vi "UseArrayOfClusterWithClasses.vi"(9 "Numeric 3":dbl=33.0, 10 "Numeric 2":dbl=22.0, 11 "Numeric":dbl=11.0) -> (3 "output array":T1(array[cluster]))   [LabVIEW 2013]
uses:
  ClassDefinitions/SimpleClassWithProperties/myClass.lvclass
panel:
  in  "array":T1(array[cluster])
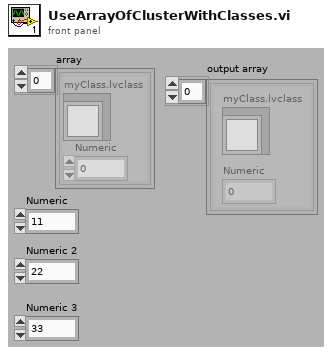
[diagram p1: front panel]
types:
  T1 = cluster{"myClass.lvclass":refnum<class "myClass.lvclass">, "Numeric":dbl}[]
  T2 = cluster{"myClass.lvclass":refnum<class "myClass.lvclass">, "Numeric":dbl}
  T3 = cluster{"myClass.lvclass":refnum<class "myClass.lvclass">, "Numeric 2":dbl}
  T4 = cluster{"myClass.lvclass":refnum<class "myClass.lvclass">, "Numeric 3":dbl}
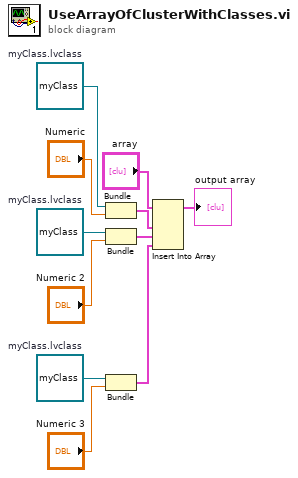
[diagram p0: block diagram]
diagram:
  w1 = refnum<class "myClass.lvclass"> refnum  # myClass.lvclass
  w2 = refnum<class "myClass.lvclass"> refnum  # myClass.lvclass
  w7 = refnum<class "myClass.lvclass"> refnum  # myClass.lvclass
  n1 = Bundle("myClass.lvclass"=w7, "Numeric"="Numeric") -> (w8:T2)  [unwired: 1 in]
  n2 = Bundle("myClass.lvclass"=w2, "Numeric 2"="Numeric 2") -> (w4:T3)  [unwired: 1 in]
  n3 = Bundle("myClass.lvclass"=w1, "Numeric 3"="Numeric 3") -> (w3:T4)  [unwired: 1 in]
  n4 = Insert Into Array(array="array", new element #1=w8, new element #2=w4, new element #3=w3) -> (→"output array":T1)  [unwired: 1 in]
